vi "Align tilt stages.vi"() -> ()   [LabVIEW 2013]
uses:
  <vilib>/Utility/file.llb/Read From Spreadsheet File (I64).vi
  <vilib>/Utility/file.llb/Write To Spreadsheet File (I64).vi
  <instrlib>/ZaberTSeries/ZaberTSeries.lvlib
panel:
  in  "Load saved position":bool=TRUE
  in  "Save position":bool=TRUE
  in  "Path for saved position":path=path "C:/Users/lab/Documents/GitHub/single-photon-vision/LabVIEW/Tools/Calibration/position.txt"
  out "Current position (RV)":i32
  out "Current position (RH)":i32
  in  "Device Number (RH)":u8=4
  in  "Device Number (RV)":u8=3
  out "Current position (LH)":i32
  in  "Device Number (LH)":u8=1
  out "Current position (LV)":i32
  out "error out":errorcluster
  in  "Step Size":i32=1000
  in  "Device Number (LV)":u8=2
  in  "error in (no error)":errorcluster
  in  "VISA resource name":refnum<visa-resource-name>="COM5"
  in  "stop":bool
  # "Press space to update from saved positions."
  # "Press space after STOP to end the VI."
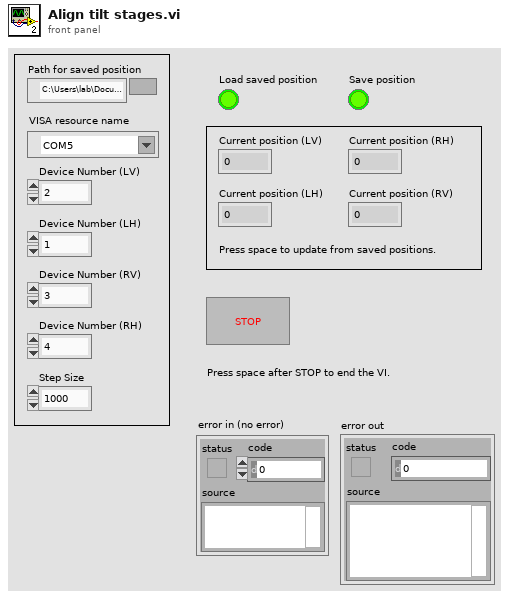
[diagram p1: front panel]
types:
  T1 = enum16{"0", "1", "2", "3", "4", "5", "6", "7", "8", "9", "A", "B", "C", "D", "E", "F", "G", "H", "I", "J", "K", "L", "M", "N", "O", "P", "Q", "R", "S", "T", "U", "V", "W", "X", "Y", "Z", "F1", "F2", "F3", "F4", "F5", "F6", "F7", "F8", "F9", "F10", "F11", "F12", "F13", "F14", "F15", "ADD", "BACK", "BACKSLASH", "CAPITAL", "COMMA", "DECIMAL", "DELETE", "DIVIDE", "DOWN", "END", "EQUALS", "ESCAPE", "GRAVE (`)", "HOME", "INSERT", "LBRACKET", "LCONTROL", "LEFT", "L ALT", "LSHIFT", "LWIN", "MINUS", "MULTIPLY", "NEXT", "NUMLOCK", "NUMPAD_0", "NUMPAD_1", "NUMPAD_2", "NUMPAD_3", "NUMPAD_4", "NUMPAD_5", "NUMPAD_6", "NUMPAD_7", "NUMPAD_8", "NUMPAD_9", "PAUSE", "PERIOD", "PRIOR (PG UP)", "RBRACKET", "RCONTROL", "RETURN", "RIGHT", "R ALT", "RSHIFT", "RWIN", "SCROLL", "SEMICOLON", "SLASH", "SPACE", "SUBTRACT", "TAB", "UP", "ENTER (num pad)", "' (quote)"}
  T2 = cluster{"Response Count":i32, "Command":u8, "Response Count":i32, "Response Count":i32}
  T3 = typedef "ZaberTSeries.lvlib/Response.ctl" = cluster{"Device Number":u8, "Command":u8, "Data":i32}
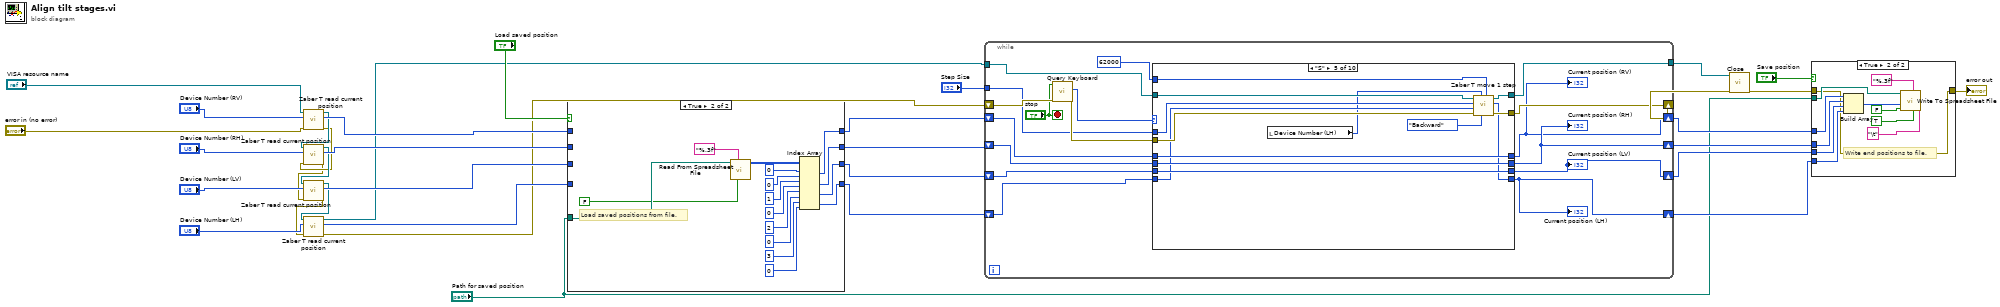
[diagram p0: block diagram]
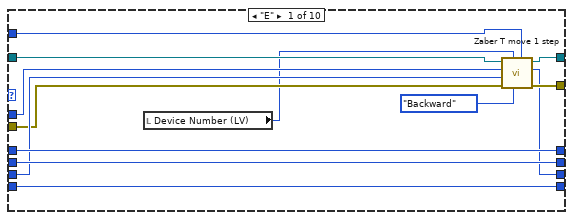
[diagram p4: hidden frame]
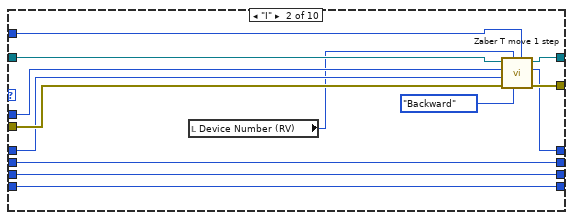
[diagram p5: hidden frame]
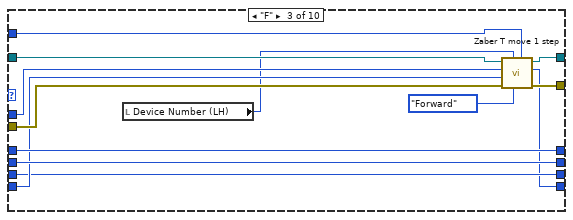
[diagram p6: hidden frame]
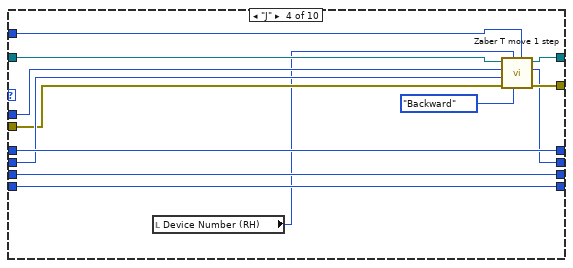
[diagram p7: hidden frame]
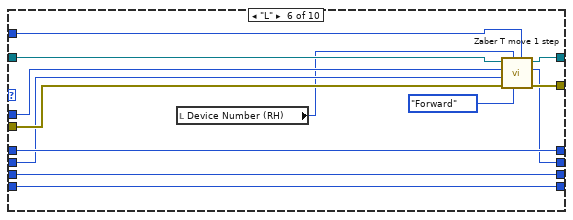
[diagram p8: hidden frame]
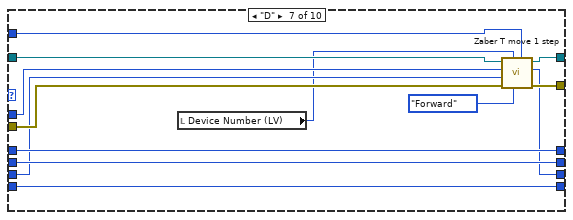
[diagram p9: hidden frame]
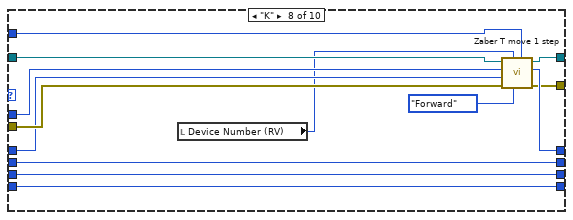
[diagram p10: hidden frame]
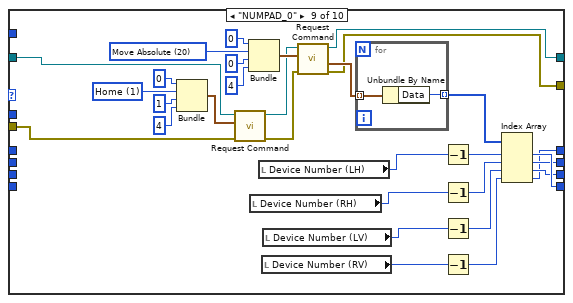
[diagram p11: hidden frame]
diagram:
  n1 = call "Zaber T read current position.vi"("error in (no error)"="error in (no error)", "Device Number (LV)"="Device Number (RV)", "VISA Refnum in"="VISA resource name") -> ("error out"=w4:errorcluster, "Current position (LV)"=w13:i32, "VISA Refnum out"=w9:refnum<visa-resource-name>)  [unwired: 6 in]
  n2 = call "Zaber T read current position.vi"("error in (no error)"=w4, "Device Number (LV)"="Device Number (RH)", "VISA Refnum in"=w9) -> ("error out"=w3:errorcluster, "Current position (LV)"=w11:i32, "VISA Refnum out"=w8:refnum<visa-resource-name>)  [unwired: 6 in]
  n3 = call "Zaber T read current position.vi"("error in (no error)"=w3, "Device Number (LV)"="Device Number (LV)", "VISA Refnum in"=w8) -> ("error out"=w2:errorcluster, "Current position (LV)"=w20:i32, "VISA Refnum out"=w7:refnum<visa-resource-name>)  [unwired: 6 in]
  n4 = call "Zaber T read current position.vi"("error in (no error)"=w2, "Device Number (LV)"="Device Number (LH)", "VISA Refnum in"=w7) -> ("error out"=w1:errorcluster, "Current position (LV)"=w15:i32, "VISA Refnum out"=w6:refnum<visa-resource-name>)  [unwired: 6 in]
  n5 = case shown="True" "Load saved position" {
    tunnel: "Path for saved position" -> [_ w54]
    tunnel: w13 -> [w38 _]
    tunnel: [w38 w43] -> w21
    tunnel: w20 -> [w37 _]
    tunnel: [w37 w41] -> w19
    tunnel: [w36 w40] -> w18
    tunnel: w15 -> [w36 _]
    tunnel: [w35 w42] -> w17
    tunnel: w11 -> [w35 _]
    frame False {
    }
    frame True {
      # "Load saved positions from file."
      n6 = call-poly <vilib>:"Read From Spreadsheet File.vi"("transpose (no:F)"=FALSE, "format (%d)"="%.3f" ("format (%.3f)"), "file path (dialog if empty)"=w54) -> ("all rows"=w39:i64[][])  [unwired: 4 in, 4 out]
      n7 = Index Array(array=w39, index (row) #1=0 ("index"), index (col) #1=0 ("disabled index (col)"), index (row) #2=1 ("index"), index (col) #2=0 ("disabled index (col)"), index (row) #3=2 ("index"), index (col) #3=0 ("disabled index (col)"), index (row) #4=3 ("index"), index (col) #4=0 ("disabled index (col)")) -> (element #1=w43:i64, element #2=w42:i64, element #3=w41:i64, element #4=w40:i64)
    }
  }
  n8 = while {
    shift-right: [w69] -> w33
    shift-left: w1 -> [w71]
    tunnel: "Step Size" -> [w67]
    tunnel: w6 -> [w66]
    tunnel: [w65] -> w31
    shift-right: [w64] -> w28
    shift-left: w19 -> [w60]
    shift-right: [w62] -> w27
    shift-left: w18 -> [w61]
    shift-right: [w58] -> w29
    shift-left: w17 -> [w57]
    shift-right: [w56] -> w30
    shift-left: w21 -> [w59]
    stop <- "stop" stop-if-true
    n9 = call "Query Keyboard.vi"("error in (no error)"=w71, "Stop?"="stop") -> ("error out"=w70:errorcluster, "element"=w68:T1)  [unwired: 8 in]
    n10 = case shown="\"S\"" w68 {
      tunnel: w70 -> [w77 w94 w107 w118 w133 w145 w158 w172 w201 w213]
      tunnel: [w76 w97 w102 w117 w132 w140 w152 w165 w182 w213] -> w69
      tunnel: w66 -> [w81 w96 w99 w122 w129 w142 w155 w171 w202 w212]
      tunnel: w67 -> [w79 w93 w105 w119 w126 w143 w156 w169 _ _]
      tunnel: [w75 w95 w103 w116 w130 w139 w153 w164 w180 w212] -> w65
      tunnel: [w74 w88 w101 w113 w134 w147 w151 w173 w192 w211] -> w64
      tunnel: w60 -> [w78 w88 w101 w113 w134 w147 w157 w173 _ w211]
      tunnel: 62000 ("Data") -> [w80 w87 w106 w120 w128 w146 w154 w170 _ _]
      tunnel: [w84 w92 w100 w112 w131 w148 w162 w175 w197 w210] -> w62
      tunnel: w61 -> [w84 w92 w104 w112 w127 w148 w162 w175 _ w210]
      tunnel: w59 -> [w82 w89 w109 w123 w135 w149 w160 w167 _ w208]
      tunnel: [w83 w91 w110 w115 w136 w138 w161 w174 w194 w209] -> w58
      tunnel: w57 -> [w83 w91 w110 w121 w136 w144 w161 w174 _ w209]
      tunnel: [w82 w90 w109 w123 w135 w149 w160 w168 w190 w208] -> w56
      frame "E" {
        n11 = local read "Device Number (LV)"() -> (w72:u8)
        n12 = call "Zaber T move 1 step.vi"("Maximum"=w80, "Direction"=enum16{"Forward", "Backward"}."Backward", "Device Number"=w72, "error in (no error)"=w77, "Current position in"=w78, "Step Size"=w79, "VISA Refnum in"=w81) -> ("error out"=w76:errorcluster, "Current position out"=w74:i64, "VISA Refnum out"=w75:refnum<visa-resource-name>)  [unwired: 2 in]
      }
      frame "I" {
        n13 = local read "Device Number (RV)"() -> (w85:u8)
        n14 = call "Zaber T move 1 step.vi"("Maximum"=w87, "Direction"=enum16{"Forward", "Backward"}."Backward", "Device Number"=w85, "error in (no error)"=w94, "Current position in"=w89, "Step Size"=w93, "VISA Refnum in"=w96) -> ("error out"=w97:errorcluster, "Current position out"=w90:i64, "VISA Refnum out"=w95:refnum<visa-resource-name>)  [unwired: 2 in]
      }
      frame "F" {
        n15 = local read "Device Number (LH)"() -> (w98:u8)
        n16 = call "Zaber T move 1 step.vi"("Maximum"=w106, "Direction"=enum16{"Forward", "Backward"}."Forward", "Device Number"=w98, "error in (no error)"=w107, "Current position in"=w104, "Step Size"=w105, "VISA Refnum in"=w99) -> ("error out"=w102:errorcluster, "Current position out"=w100:i64, "VISA Refnum out"=w103:refnum<visa-resource-name>)  [unwired: 2 in]
      }
      frame "J" {
        n17 = local read "Device Number (RH)"() -> (w111:u8)
        n18 = call "Zaber T move 1 step.vi"("Maximum"=w120, "Direction"=enum16{"Forward", "Backward"}."Backward", "Device Number"=w111, "error in (no error)"=w118, "Current position in"=w121, "Step Size"=w119, "VISA Refnum in"=w122) -> ("error out"=w117:errorcluster, "Current position out"=w115:i64, "VISA Refnum out"=w116:refnum<visa-resource-name>)  [unwired: 2 in]
      }
      frame "S" {
        n19 = local read "Device Number (LH)"() -> (w124:u8)
        n20 = call "Zaber T move 1 step.vi"("Maximum"=w128, "Direction"=enum16{"Forward", "Backward"}."Backward", "Device Number"=w124, "error in (no error)"=w133, "Current position in"=w127, "Step Size"=w126, "VISA Refnum in"=w129) -> ("error out"=w132:errorcluster, "Current position out"=w131:i64, "VISA Refnum out"=w130:refnum<visa-resource-name>)  [unwired: 2 in]
      }
      frame "L" {
        n21 = local read "Device Number (RH)"() -> (w137:u8)
        n22 = call "Zaber T move 1 step.vi"("Maximum"=w146, "Direction"=enum16{"Forward", "Backward"}."Forward", "Device Number"=w137, "error in (no error)"=w145, "Current position in"=w144, "Step Size"=w143, "VISA Refnum in"=w142) -> ("error out"=w140:errorcluster, "Current position out"=w138:i64, "VISA Refnum out"=w139:refnum<visa-resource-name>)  [unwired: 2 in]
      }
      frame "D" {
        n23 = local read "Device Number (LV)"() -> (w150:u8)
        n24 = call "Zaber T move 1 step.vi"("Maximum"=w154, "Direction"=enum16{"Forward", "Backward"}."Forward", "Device Number"=w150, "error in (no error)"=w158, "Current position in"=w157, "Step Size"=w156, "VISA Refnum in"=w155) -> ("error out"=w152:errorcluster, "Current position out"=w151:i64, "VISA Refnum out"=w153:refnum<visa-resource-name>)  [unwired: 2 in]
      }
      frame "K" {
        n25 = local read "Device Number (RV)"() -> (w163:u8)
        n26 = call "Zaber T move 1 step.vi"("Maximum"=w170, "Direction"=enum16{"Forward", "Backward"}."Forward", "Device Number"=w163, "error in (no error)"=w172, "Current position in"=w167, "Step Size"=w169, "VISA Refnum in"=w171) -> ("error out"=w165:errorcluster, "Current position out"=w168:i64, "VISA Refnum out"=w164:refnum<visa-resource-name>)  [unwired: 2 in]
      }
      frame "NUMPAD_0" {
        w187 = u8 20 items=["Echo"=55, "Home"=1, "Move Absolute"=20, "Move Relative"=21, "Move at Constant Speed"=22, "Renumber"=2, "Restore Settings"=36, "Stop"=23] ("Command")
        w203 = u8 1 items=["Echo"=55, "Home"=1, "Move Absolute"=20, "Move Relative"=21, "Move at Constant Speed"=22, "Renumber"=2, "Restore Settings"=36, "Stop"=23] ("Command")
        n27 = Bundle("Response Count"=0, "Command"=w203, "Response Count"=1, "Response Count"=4) -> (w205:T2)  [unwired: 1 in]
        n28 = call <instrlib>:"Request Command.vi"("error in (no error)"=w201, "Request"=w205, "VISA resource name"=w202) -> ("error out"=w183:errorcluster, "VISA resource name out"=w181:refnum<visa-resource-name>)  [unwired: 5 in, 2 out]
        n29 = Bundle("Response Count"=0, "Command"=w187, "Response Count"=0, "Response Count"=4) -> (w189:T2)  [unwired: 1 in]
        n30 = local read "Device Number (RH)"() -> (w178:u8)
        n31 = local read "Device Number (LH)"() -> (w179:u8)
        n32 = local read "Device Number (RV)"() -> (w176:u8)
        n33 = local read "Device Number (LV)"() -> (w177:u8)
        n34 = call <instrlib>:"Request Command.vi"("error in (no error)"=w183, "Request"=w189, "VISA resource name"=w181) -> ("error out"=w182:errorcluster, "Responses out"=w184:T3[], "VISA resource name out"=w180:refnum<visa-resource-name>)  [unwired: 5 in, 1 out]
        n35 = for {
          tunnel: w184 -> [w207] mode=indexing
          tunnel: [w206] -> w198 mode=indexing
          n36 = Unbundle By Name(w207) -> ("Data"=w206:i32)
        }
        n37 = Decrement(x=w179) -> (x-1=w196:u8)
        n38 = Decrement(x=w178) -> (x-1=w195:u8)
        n39 = Decrement(x=w177) -> (x-1=w193:u8)
        n40 = Decrement(x=w176) -> (x-1=w191:u8)
        n41 = Index Array(array=w198, index #1=w196, index #2=w195, index #3=w193, index #4=w191) -> (element #1=w197:i32, element #2=w194:i32, element #3=w192:i32, element #4=w190:i32)
      }
      frame "SPACE", Default {
      }
    }
    "Current position (LV)" <- w64
    "Current position (LH)" <- w62
    "Current position (RH)" <- w58
    "Current position (RV)" <- w56
  }
  n42 = call <instrlib>:"Close.vi"("error in (no error)"=w33, "VISA resource name"=w31) -> ("error out"=w26:errorcluster)  [unwired: 8 in, 1 out]
  n43 = case shown="True" "Save position" {
    tunnel: w30 -> [_ w225]
    tunnel: w29 -> [_ w224]
    tunnel: w28 -> [_ w223]
    tunnel: w27 -> [_ w222]
    tunnel: "Path for saved position" -> [_ w221]
    tunnel: w26 -> [w214 w215]
    tunnel: [w214 w215] -> w25
    frame False {
    }
    frame True {
      # "Write end positions to file."
      n44 = Build Array(w225, w224, w223, w222) -> (w216:i64[])
      n45 = call-poly <vilib>:"Write To Spreadsheet File.vi"("delimiter (\\t)"="\t" ("delimiter (\\t)"), "transpose? (no:F)"=TRUE, "format (%d)"="%.3f" ("format (%.3f)"), "append to file? (new file:F)"=FALSE, "1D data"=w216, "file path (dialog if empty)"=w221) -> ()  [unwired: 2 in, 1 out]
    }
  }
  "error out" <- w25
